vi "long_cmd_read.vi"(4 "data":u8[](array[numeric]), 5 "COM":bool, 6 "dwLen":u32, 7 "VISA name":refnum<visa-resource-name>, 8 "error in":errorcluster, 9 "dwAddr2":u32, 10 "dwAddr1":u32, 11 "vd_cmd_long_header_t":T1) -> (0 "error out":errorcluster, 2 "data out":u8[](array[numeric]), 3 "return":i32)   [LabVIEW 2016]
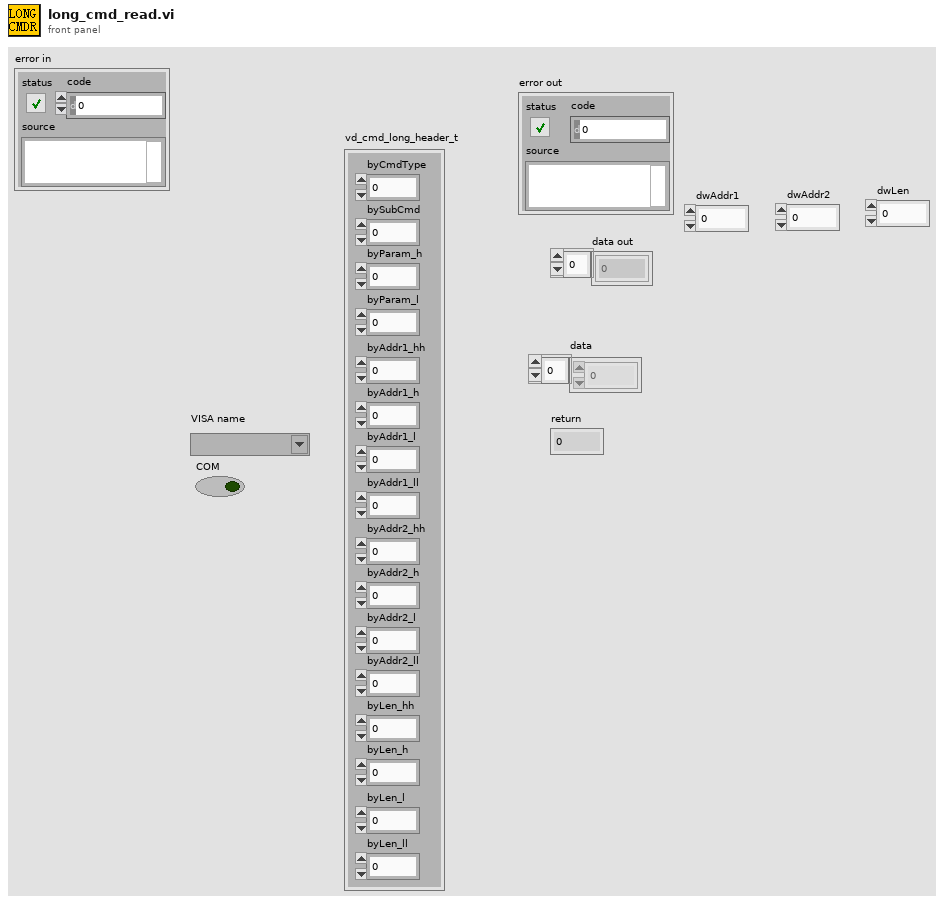
[diagram p1: front panel]
types:
  T1 = cluster{"byCmdType":u8, "bySubCmd":u8, "byParam_h":u8, "byParam_l":u8, "byAddr1_hh":u8, "byAddr1_h":u8, "byAddr1_l":u8, "byAddr1_ll":u8, "byAddr2_hh":u8, "byAddr2_h":u8, "byAddr2_l":u8, "byAddr2_ll":u8, "byLen_hh":u8, "byLen_h":u8, "byLen_l":u8, "byLen_ll":u8}
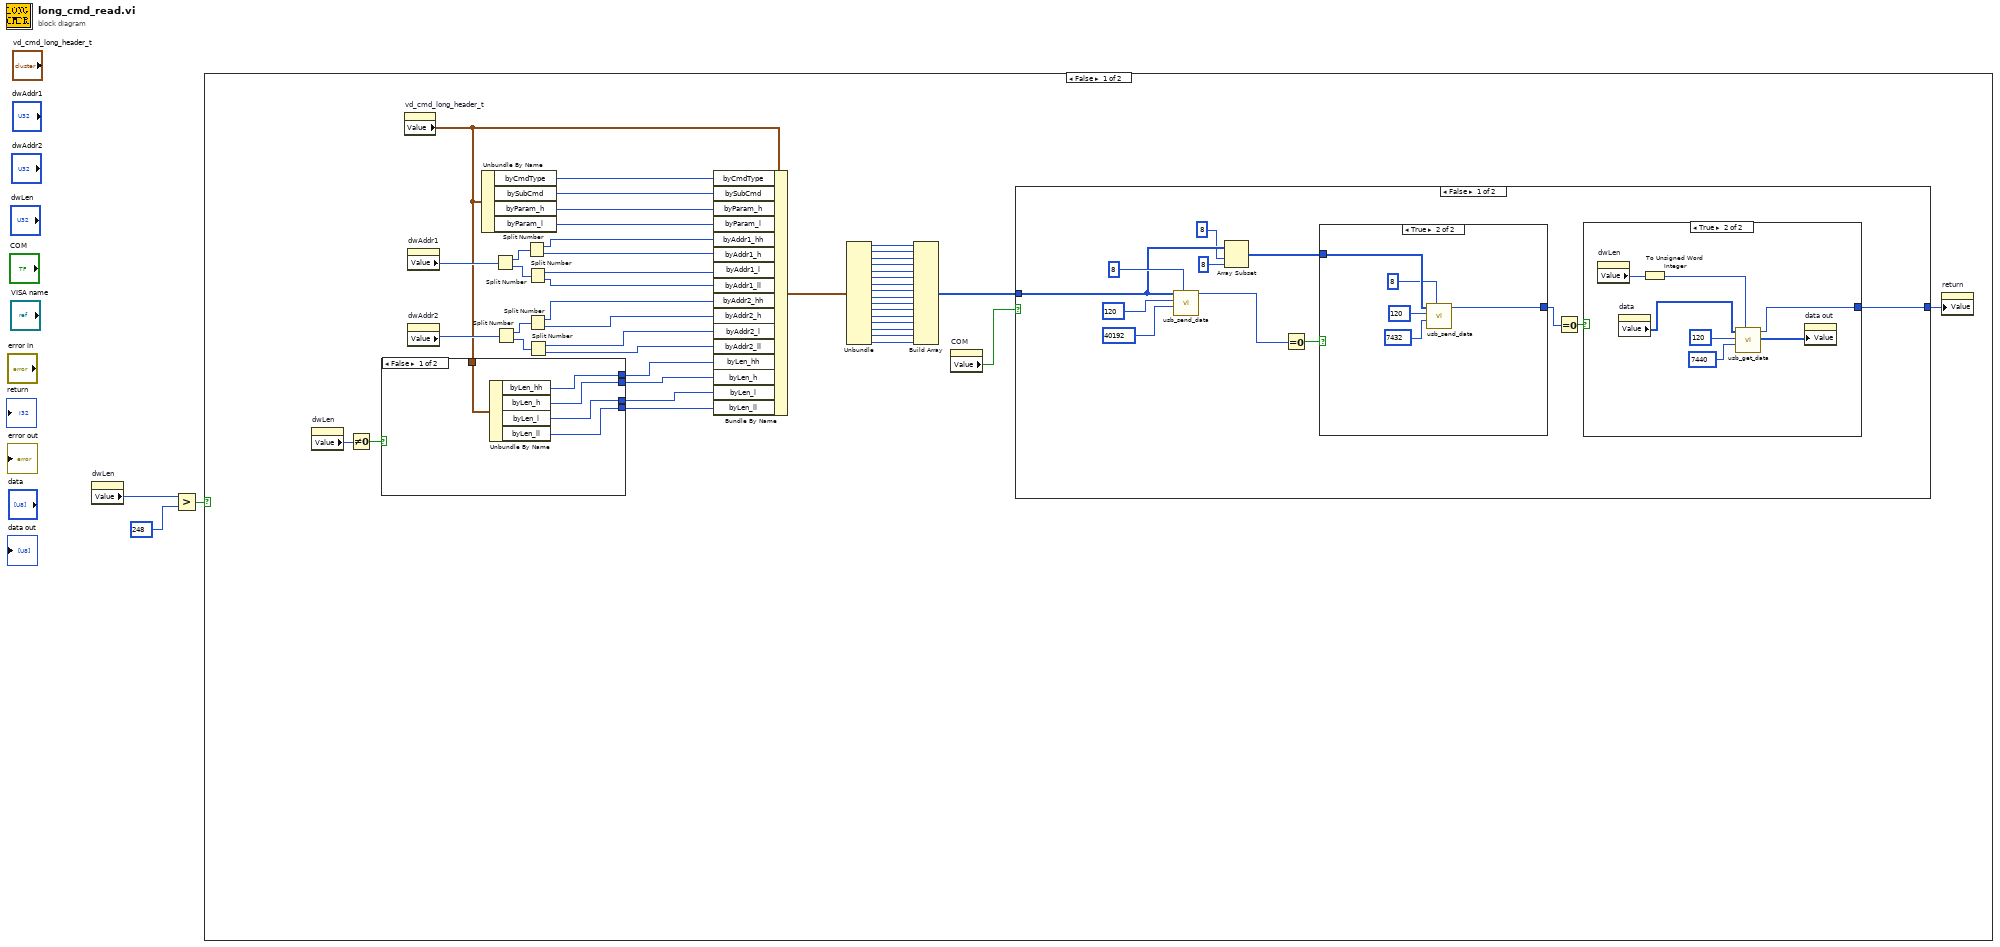
[diagram p0: block diagram]
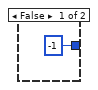
[diagram p2: hidden frame]
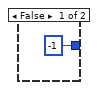
[diagram p3: hidden frame]
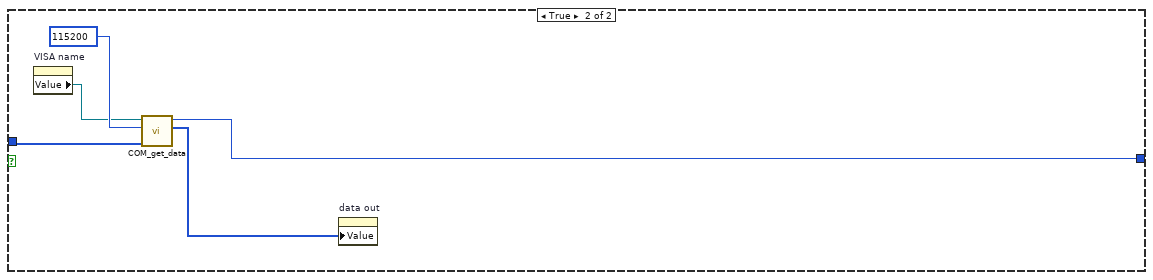
[diagram p4: hidden frame]
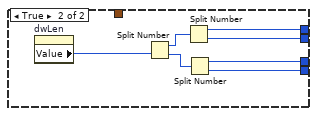
[diagram p5: hidden frame]
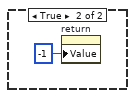
[diagram p6: hidden frame]
diagram:
  n1 = property on="dwLen" class="DigNum (strict)"() -> ("Value"=w2:u32)  [unwired: 2 in, 2 out]
  n2 = Greater?(x=w2, y=u32 248) -> (0:w3:bool)
  n3 = case shown="False" w3 {
    frame False {
      n4 = property on="dwLen" class="DigNum (strict)"() -> ("Value"=w48:u32)  [unwired: 2 in, 2 out]
      n5 = Not Equal To 0?(x=w48) -> (x != 0?=w25:bool)
      n6 = property on="vd_cmd_long_header_t" class="Clust (strict)"() -> ("Value"=w24:T1)  [unwired: 2 in, 2 out]
      n7 = case shown="False" w25 {
        tunnel: [w83 w88] -> w29
        tunnel: [w82 w87] -> w28
        tunnel: [w81 w86] -> w27
        tunnel: [w80 w85] -> w26
        tunnel: w24 -> [w84 _]
        frame False {
          n8 = Unbundle By Name(w84) -> ("byLen_hh"=w83:u8, "byLen_h"=w82:u8, "byLen_l"=w81:u8, "byLen_ll"=w80:u8)
        }
        frame True {
          n9 = property on="dwLen" class="DigNum (strict)"() -> ("Value"=w89:u32)  [unwired: 2 in, 2 out]
          n10 = Split Number(x=w89) -> (hi(x)=w91:u16, lo(x)=w90:u16)
          n11 = Split Number(x=w91) -> (hi(x)=w88:u8, lo(x)=w87:u8)
          n12 = Split Number(x=w90) -> (hi(x)=w86:u8, lo(x)=w85:u8)
        }
      }
      n13 = property on="dwAddr1" class="DigNum (strict)"() -> ("Value"=w45:u32)  [unwired: 2 in, 2 out]
      n14 = property on="dwAddr2" class="DigNum (strict)"() -> ("Value"=w42:u32)  [unwired: 2 in, 2 out]
      n15 = Unbundle By Name(w24) -> ("byCmdType"=w41:u8, "bySubCmd"=w40:u8, "byParam_h"=w39:u8, "byParam_l"=w38:u8)
      n16 = Split Number(x=w45) -> (hi(x)=w47:u16, lo(x)=w46:u16)
      n17 = Split Number(x=w42) -> (hi(x)=w43:u16, lo(x)=w44:u16)
      n18 = Split Number(x=w47) -> (hi(x)=w37:u8, lo(x)=w36:u8)
      n19 = Split Number(x=w46) -> (hi(x)=w35:u8, lo(x)=w34:u8)
      n20 = Split Number(x=w43) -> (hi(x)=w33:u8, lo(x)=w32:u8)
      n21 = Split Number(x=w44) -> (hi(x)=w31:u8, lo(x)=w30:u8)
      n22 = Bundle By Name(cluster=w24, "byCmdType"=w41, "bySubCmd"=w40, "byParam_h"=w39, "byParam_l"=w38, "byAddr1_hh"=w37, "byAddr1_h"=w36, "byAddr1_l"=w35, "byAddr1_ll"=w34, "byAddr2_hh"=w33, "byAddr2_h"=w32, "byAddr2_l"=w31, "byAddr2_ll"=w30, "byLen_hh"=w29, "byLen_h"=w28, "byLen_l"=w27, "byLen_ll"=w26) -> (w23:T1)
      n23 = Unbundle(w23) -> ("byCmdType"=w22:u8, "bySubCmd"=w21:u8, "byParam_h"=w20:u8, "byParam_l"=w19:u8, "byAddr1_hh"=w18:u8, "byAddr1_h"=w17:u8, "byAddr1_l"=w16:u8, "byAddr1_ll"=w15:u8, "byAddr2_hh"=w14:u8, "byAddr2_h"=w13:u8, "byAddr2_l"=w12:u8, "byAddr2_ll"=w11:u8, "byLen_hh"=w10:u8, "byLen_h"=w9:u8, "byLen_l"=w8:u8, "byLen_ll"=w7:u8)
      n24 = Build Array(w22, w21, w20, w19, w18, w17, w16, w15, w14, w13, w12, w11, w10, w9, w8, w7) -> (w5:u8[])
      n25 = property on="COM" class="Bool (strict)"() -> ("Value"=w6:bool)  [unwired: 2 in, 2 out]
      n26 = case shown="False" w6 {
        tunnel: w5 -> [w55 w77]
        tunnel: [w49 w76] -> w4
        frame False {
          n27 = call "usb_send_data.vi"("byVdCmdHeaderLen"=u16 8, "I2C_VD_BUFFER_RW"=u16 40192, "I2C_SLAVE_ID"=u8 120, "data"=w55) -> ("return"=w56:i32)  [unwired: 6 in, 1 out]
          n28 = Array Subset(array=w55, index=8, length=8) -> (w52:u8[])
          n29 = Equal To 0?(x=w56) -> (x = 0?=w57:bool)
          n30 = case shown="True" w57 {
            tunnel: w52 -> [_ w74]
            tunnel: [-1 ("return") w70] -> w50
            frame False {
            }
            frame True {
              n31 = call "usb_send_data.vi"("byVdCmdHeaderLen"=u16 8, "I2C_VD_BUFFER_RW"=u16 7432, "I2C_SLAVE_ID"=u8 120, "data"=w74) -> ("return"=w70:i32)  [unwired: 6 in, 1 out]
            }
          }
          n32 = Equal To 0?(x=w50) -> (x = 0?=w51:bool)
          n33 = case shown="True" w51 {
            tunnel: [-1 ("return") w64] -> w49
            frame False {
            }
            frame True {
              n34 = property on="dwLen" class="DigNum (strict)"() -> ("Value"=w67:u32)  [unwired: 2 in, 2 out]
              n35 = property on="data" class="Arr (strict)"() -> ("Value"=w62:u8[])  [unwired: 2 in, 2 out]
              n36 = To Unsigned Word Integer(number=w67) -> (unsigned 16bit integer=w65:u16)
              n37 = call "usb_get_data.vi"("byVdCmdHeaderLen"=w65, "I2C_VD_BUFFER_RW"=u16 7440, "I2C_SLAVE_ID"=u8 120, "data"=w62) -> ("data out"=w63:u8[], "return"=w64:i32)  [unwired: 5 in, 1 out]
              n38 = property on="data out" class="Arr (strict)"("Value"=w63) -> ()  [unwired: 2 in, 2 out]
            }
          }
        }
        frame True {
          n39 = property on="VISA name" class="VISAName"() -> ("Value"=w78:refnum<visa-resource-name>)  [unwired: 2 in, 2 out]
          n40 = call "COM_get_data.vi"("data"=w77, "baud rate (9600)"=u32 115200, "VISA name"=w78) -> ("data out"=w75:u8[], "return"=w76:i32)  [unwired: 7 in]
          n41 = property on="data out" class="Arr (strict)"("Value"=w75) -> ()  [unwired: 2 in, 2 out]
        }
      }
      n42 = property on="return" class="DigNum (strict)"("Value"=w4) -> ()  [unwired: 2 in, 2 out]
    }
    frame True {
      n43 = property on="return" class="DigNum (strict)"("Value"=-1 ("return")) -> ()  [unwired: 2 in, 2 out]
    }
  }
